vi "Set Waveform Definition.vi"(8 "error in (no error)":errorcluster, 10 "Waveform Definition":T1, 11 "Signal Generator in":refnum<class "Signal Generator.lvclass">) -> (0 "error out":errorcluster, 3 "Signal Generator out":refnum<class "Signal Generator.lvclass">)   [LabVIEW 2020, in "Signal Generator.lvlib" / "Signal Generator.lvclass"]
uses:
  Signal Generator.lvclass
  Waveform Definition.ctl
  Waveform Type.ctl
  Signal Generator.lvclass/Signal Generator.ctl
  build/ppl/lv-hal.lvlibp/Device/Device.lvclass
  C:/dev/HAL Demo/build/ppl/lv-hal.lvlibp/Device/Device.lvclass
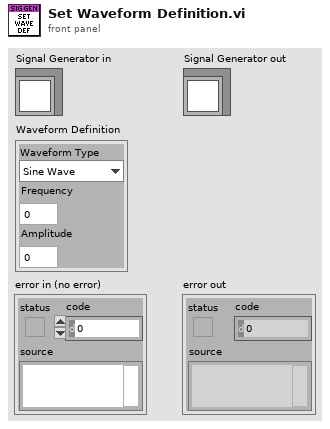
[diagram p1: front panel]
types:
  T1 = typedef "Signal Generator.lvlib/Signal Generator.lvclass/Waveform Definition.ctl" = cluster{"Waveform Type":T2, "Frequency":dbl, "Amplitude":dbl}
  T2 = typedef "Signal Generator.lvlib/Signal Generator.lvclass/Waveform Type.ctl" = enum16{"Sine Wave", "Triangle Wave", "Square Wave", "Sawtooth Wave"}
  T3 = typedef "Signal Generator.lvlib/Signal Generator.lvclass/Ref Data.ctl" = cluster{"Waveform Definition":T1}
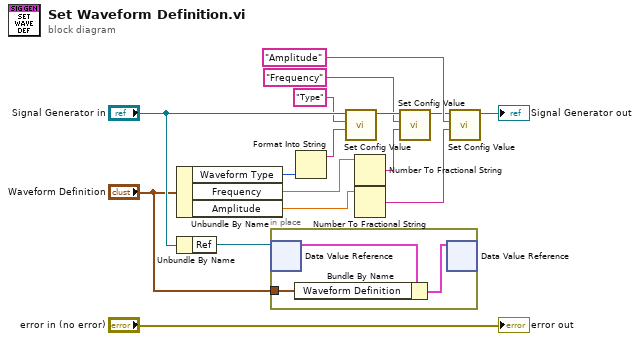
[diagram p0: block diagram]
diagram:
  n1 = Unbundle By Name("Waveform Definition") -> ("Waveform Type"=w11:T2, "Frequency"=w8:dbl, "Amplitude"=w2:dbl)
  n2 = Unbundle By Name("Signal Generator in") -> ("Ref"=w15:refnum<data-value>)
  n3 = in-place {
    in-place-border: "Waveform Definition" -> [w17]
    n4 = in-place-dvr #1(w15) -> (w19:T3)  [unwired: 1 out]
    n5 = Bundle By Name(cluster=w19, "Waveform Definition"=w17) -> (w18:T3)
    n6 = in-place-dvr #1(w18) -> ()  [unwired: 2 out]
  }
  n7 = Format Into String(w11) -> (resulting string=w10:string)  [unwired: 3 in, 1 out]
  n8 = call "Set Config Value.vi"("Value"=w10, "Config Key"="Type", "Device in"="Signal Generator in") -> ("Device out"=w9:refnum<class "Signal Generator.lvclass">)  [unwired: 7 in, 1 out]
  n9 = Number To Fractional String(number=w8) -> (F-format string=w3:string)  [unwired: 3 in]
  n10 = Number To Fractional String(number=w2) -> (F-format string=w1:string)  [unwired: 3 in]
  n11 = call "Set Config Value.vi"("Value"=w3, "Config Key"="Frequency", "Device in"=w9) -> ("Device out"=w5:refnum<class "Signal Generator.lvclass">)  [unwired: 7 in, 1 out]
  n12 = call "Set Config Value.vi"("Value"=w1, "Config Key"="Amplitude", "Device in"=w5) -> ("Device out"=→"Signal Generator out":refnum<class "Signal Generator.lvclass">)  [unwired: 7 in, 1 out]
  "error out" <- "error in (no error)"
